vi "Untitled 33.vi"() -> ()   [LabVIEW 2020]
uses:
  forms AF/Autoclose manager/Form ID.ctl
  forms AF/Autoclose manager/Form State.ctl
  forms AF/Open Close Logic Simple Table/Open Close Logic Simple Table.lvclass
  forms AF/Form Server Managers.lvlib
panel:
  out "Nested 2":T1[](array[typedef])
  out "Caller 2":T1[](array[typedef])
  out "Nested":T1[](array[typedef])
  out "Caller":T1[](array[typedef])
  out "Close Nested":T1[](array[typedef])
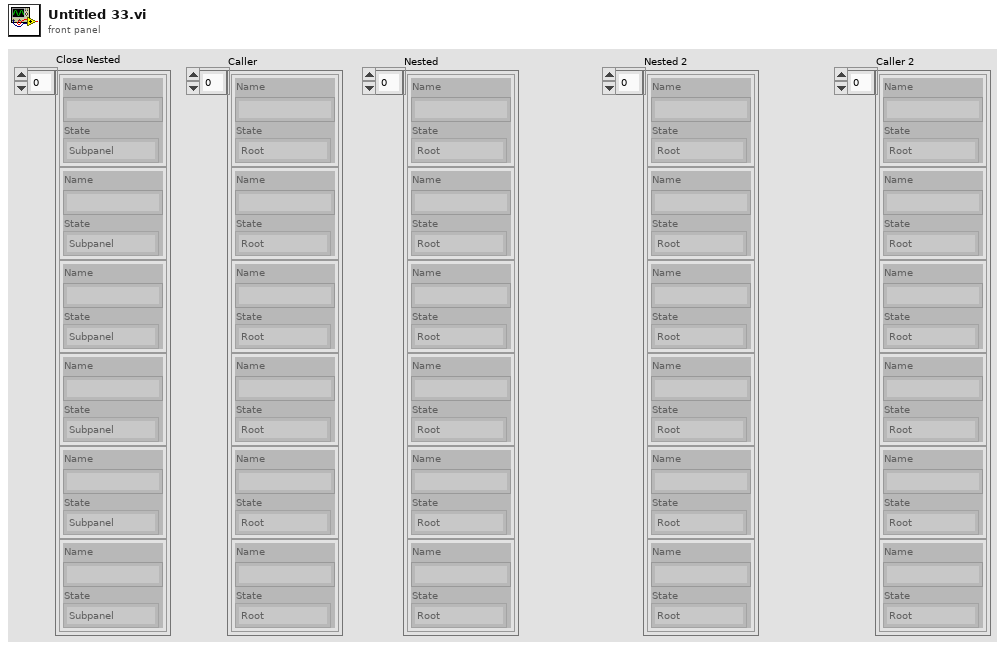
[diagram p1: front panel]
types:
  T1 = typedef "Form Server Managers.lvlib/Form ID.ctl" = cluster{"Name":string, "State":T2}
  T2 = typedef "Form Server Managers.lvlib/Form State.ctl" = enum16{"Root", "Subpanel", "Window"}
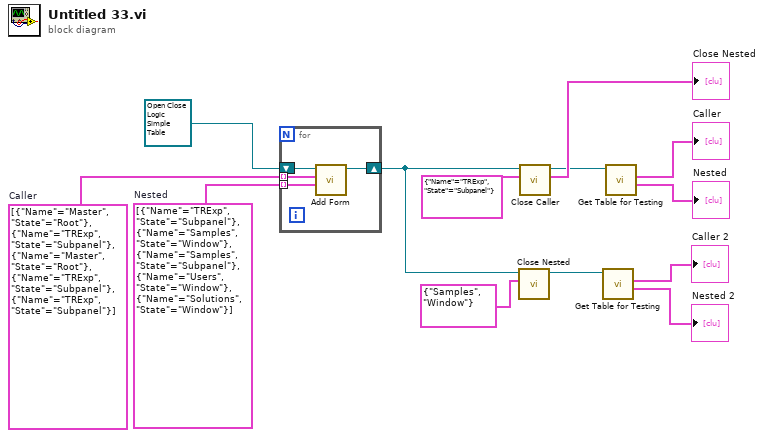
[diagram p0: block diagram]
diagram:
  w12 = T1[] [{"Name"="TRExp", "State"=enum."Subpanel"}, {"Name"="Samples", "State"=enum."Window"}, {"Name"="Samples", "State"=enum."Subpanel"}, {"Name"="Users", "State"=enum."Window"}, {"Name"="Solutions", "State"=enum."Window"}]  # Nested
  w13 = T1[] [{"Name"="Master", "State"=enum."Root"}, {"Name"="TRExp", "State"=enum."Subpanel"}, {"Name"="Master", "State"=enum."Root"}, {"Name"="TRExp", "State"=enum."Subpanel"}, {"Name"="TRExp", "State"=enum."Subpanel"}]  # Caller
  n1 = for {
    tunnel: w13 -> [w17] mode=indexing
    tunnel: w12 -> [w16] mode=indexing
    shift-right: [w15] -> w11
    shift-left: refnum<class "Open Close Logic Simple Table.lvclass"> refnum ("Open Close Logic Simple Table.lvlib:Open Close Logic Simple Table.lvclass") -> [w14]
    n2 = call-dynamic "Add Form.vi"("Nested"=w16, "Caller"=w17, "Autoclose manager in"=w14) -> ("Autoclose manager out"=w15:refnum<class "Open Close Logic Simple Table.lvclass">)  [unwired: 6 in, 2 out]
  }
  n3 = call-dynamic "Close Nested.vi"("Nested"=T1 {"Name"="Samples", "State"=enum."Window"}, "Open Close Logic Simple Table in"=w11) -> ("Open Close Logic Simple Table out"=w3:refnum<class "Open Close Logic Simple Table.lvclass">)  [unwired: 8 in, 1 out]
  n4 = call-dynamic "Close Caller.vi"("Caller"=T1 {"Name"="TRExp", "State"=enum."Subpanel"}, "Open Close Logic Simple Table in"=w11) -> ("Close Nested"=→"Close Nested":T1[], "Open Close Logic Simple Table out"=w6:refnum<class "Open Close Logic Simple Table.lvclass">)  [unwired: 7 in, 1 out]
  n5 = call "Get Table for Testing.vi"("Open Close Logic Simple Table in"=w3) -> ("Nested"=→"Nested 2":T1[], "Caller"=→"Caller 2":T1[])  [unwired: 7 in, 2 out]
  n6 = call "Get Table for Testing.vi"("Open Close Logic Simple Table in"=w6) -> ("Nested"=→"Nested":T1[], "Caller"=→"Caller":T1[])  [unwired: 7 in, 2 out]
